vi "Dpc Get Spi.vi"(0 "hif":u32, 1 "perc":i32, 5 "cbRcv":i32, 7 "bFill":u8, 9 "rgbRcv":string, 11 "error in (no error)":errorcluster, 12 "ptrid":u16) -> (3 "perc out":i32, 4 "hif out":u32, 6 "function return":i32, 10 "rgbRcv out":string, 14 "ptrid out":u16, 15 "error out":errorcluster)   [LabVIEW 2011, in "LVH-Adept.lvlib" / "DPCUTIL.lvlib"]
doc: "DPCAPI BOOL DpcGetSpi(HANDLE hif, INT32 cbRcv, BYTE bFill, BYTE * rgbRcv, ERC * perc, TRID * ptrid);"
uses:
  DPCUTIL.lvlib
  dpcutil.dll
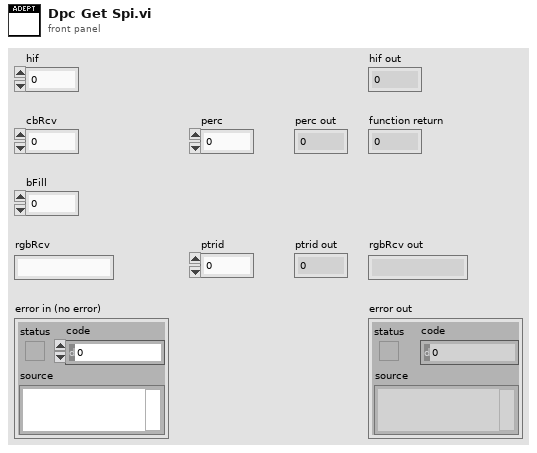
[diagram p1: front panel]
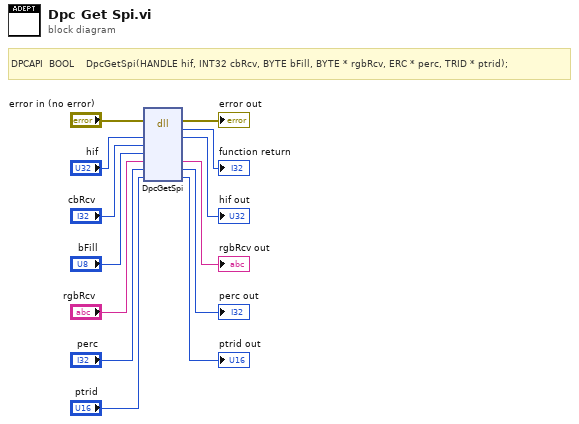
[diagram p0: block diagram]
diagram:
  # "DPCAPI  BOOL    DpcGetSpi(HANDLE hif, INT32 cbRcv, BYTE bFill, BYTE * rgbRcv, ERC * perc, TRID * ptrid);"
  n1 = dll-call lib="dpcutil.*" fn="DpcGetSpi"(error in="error in (no error)", "hif"="hif", "cbRcv"="cbRcv", "bFill"="bFill", "rgbRcv"="rgbRcv", "perc"="perc", "ptrid"="ptrid") -> (error out=→"error out":errorcluster, →"function return":i32, "hif"=→"hif out":u32, "rgbRcv"=→"rgbRcv out":string, "perc"=→"perc out":i32, "ptrid"=→"ptrid out":u16)  [unwired: 4 in, 1 out]
